vi "Set Timer Enabled.vi"(6 "Name":string, 7 "Metadata":string, 8 "error in (no error)":errorcluster, 11 "Enabled (T)":bool=TRUE) -> (0 "error out":errorcluster)   [LabVIEW 2015, in "Task Scheduler Actor API.lvclass"]
uses:
  Task Scheduler Actor API.lvclass
  Actor/Timer Config.ctl
  Re-use Libraries/Minimal Actor Framework/Messaging/Message/Message.lvclass/Message.ctl
  Globals.vi
  Re-use Libraries/Minimal Actor Framework/Messaging/Message/Message.lvclass
  Actor/Task Scheduler Actor.lvclass
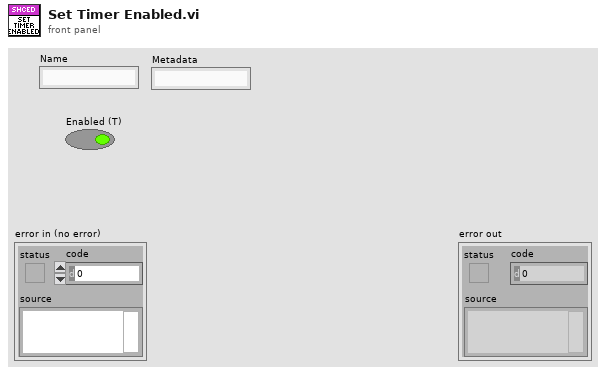
[diagram p1: front panel]
types:
  T1 = typedef "Task Scheduler Actor.lvclass/Timer Config.ctl" = cluster{"Name":string, "Period [s]":dbl, "Enabled":bool, "Metadata":string}
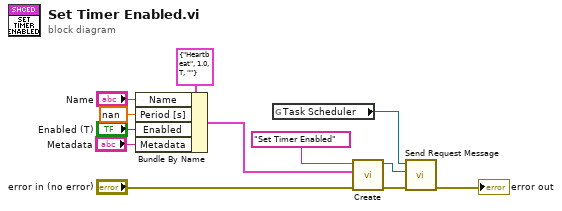
[diagram p0: block diagram]
diagram:
  n1 = Bundle By Name(cluster=T1 {"Name"="Heartbeat", "Period [s]"=1.0, "Enabled"=TRUE, "Metadata"=""} ("Timer Config"), "Name"="Name", "Period [s]"=nan, "Enabled"="Enabled (T)", "Metadata"="Metadata") -> (w5:T1)
  n2 = global read "Globals.vi" "Task Scheduler"() -> (w7:refnum<class "Task Scheduler Actor API.lvclass">)
  n3 = call "Create.vi"("error in (no error)"="error in (no error)", "Data"=w5, "Name"="Set Timer Enabled" ("Parameter")) -> ("error out"=w8:errorcluster, "Message out"=w9:refnum<class "Message.lvclass">)  [unwired: 7 in]
  n4 = call-dynamic "Send Request Message.vi"("error in (no error)"=w8, "Message"=w9, "Actor API in"=w7) -> ("error out"=→"error out":errorcluster)  [unwired: 8 in]
